vi "Write LibReader.lvclass.vi"(8 "error in (no error)":errorcluster, 10 "LibReader.lvclass":refnum<class "LibReader.lvclass">, 11 "SalProcess in":refnum<class "SalProcess.lvclass">) -> (0 "error out":errorcluster, 3 "SalProcess out":refnum<class "SalProcess.lvclass">)   [LabVIEW 2018, in "SalProcess.lvclass"]
doc: "Write the LibReader."
uses:
  SalProcess.lvclass
  LibReader/LibReader.lvclass
  SalProcess.lvclass/SalProcess.ctl
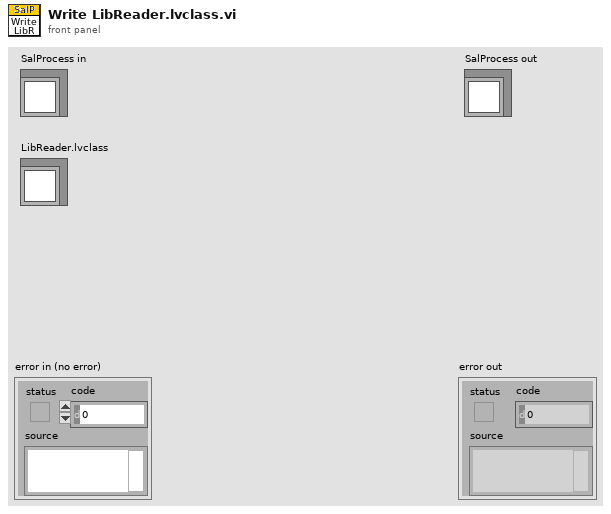
[diagram p1: front panel]
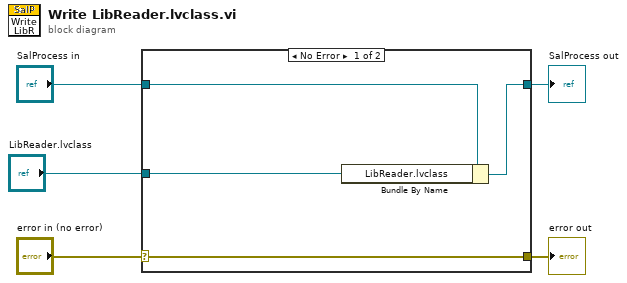
[diagram p0: block diagram]
diagram:
  n1 = case shown="No Error" "error in (no error)" {
    selector: "error in (no error)" -> [w9 w10]
    tunnel: [w9 w10] -> w4
    tunnel: [w7 w11] -> w2
    tunnel: "SalProcess in" -> [w8 w11]
    tunnel: "LibReader.lvclass" -> [w6 _]
    frame No Error {
      n2 = Bundle By Name(cluster=w8, "LibReader.lvclass"=w6) -> (w7:refnum<class "SalProcess.lvclass">)
    }
    frame Error {
    }
  }
  "error out" <- w4
  "SalProcess out" <- w2
